vi "STAGE+mono+counter_edit17.vi"() -> ()   [LabVIEW 2017]
panel:
  out "XY Graph 2":cluster{"Y":dbl[], "Y":dbl[]}[](graph)
  out "Waveform Graph 2":waveform(dbl)[](graph)
  out "Waveform Graph":waveform(dbl)[](graph)
  out "XY Graph":cluster{dbl[], dbl[]}(graph)
  out "PROGRESS":u8(slide) max=10 step=10 scale=0.0..5.0
  in  "?":enum32{"DELAY", "COUNTER", "MONO", "PLOT"}(tab)
  out "Final time [ps]":dbl
  out "Current time [ps]":dbl
  out "Initial time [ps]":dbl
  in  "Set this as t0":bool
  in  "Axis":i32=1
  in  "Motor ON":bool
  in  "Motor OFF":bool
  out "Current Position [mm]":dbl
  out "Final Position [mm]":dbl
  in  "Data Points":i32=100
  out "Current Point":i32
  in  "Step Size [um]":i32=10
  in  "Target [mm]":dbl format="%.3f"
  in  "Move":bool
  out "Initial position [mm]":dbl
  in  "GPIB address":string="23"
  in  "Count Mode":u16(ring) items=["A,B for Preset T", "A-B for Preset T", "A+B for Preset T", "A for Preset B"]
  in  "Trigger mode":u16(ring) items=["10 MHz"=0, "Input 2"=2, "Input T"=3]
  in  "Channel A Input":u16(ring)=1 items=["10 MHz", "Input 1"]
  in  "Channel B Input":u16(ring)=2 items=["Input 1"=1, "Input 2"=2]
  in  "Number of Measurements\n to take at one point/ Number of Periods":u16=1 min=1 max=2000 step=1
  in  "Time between measurements\n at one point (s)/Dwell Time":dbl=0.002 min=0.002 max=60.0 step=0.001
  in  "gate mode (CW:0)":i16(slide) scale=0.0..2.0 scale format="%.2f"
  out "Counts":i32
  in  "Integrating time \nin 10^-7 sec":dbl=10000000.0
  in  "Discriminator Level (mV)":dbl min=-300.0 max=300.0 step=0.2
  in  "Discriminator Slope":bool
  in  "Channel":i16 min=0 max=2 step=1
  out "Grating #":dbl
  out "Blaze angle":dbl
  out "Grooves/mm":dbl
  out "Mono port":T1(ring)
  out "Time delay":u32=450000 min=1
  in  "Step size":dbl=10.0 min=0.0
  in  "Scan to":i32=4000
  in  "Scan from":i32=2600
  out "Current wavelength":dbl
  in  "?":bool
  in  "Array":dbl[](array[numeric])
  out "Numeric":i32
  out "Numeric 2":i32
  out "Timeout 2":bool
  in  "?":bool
  out "Timeout":bool
  in  "Collect Data!":bool
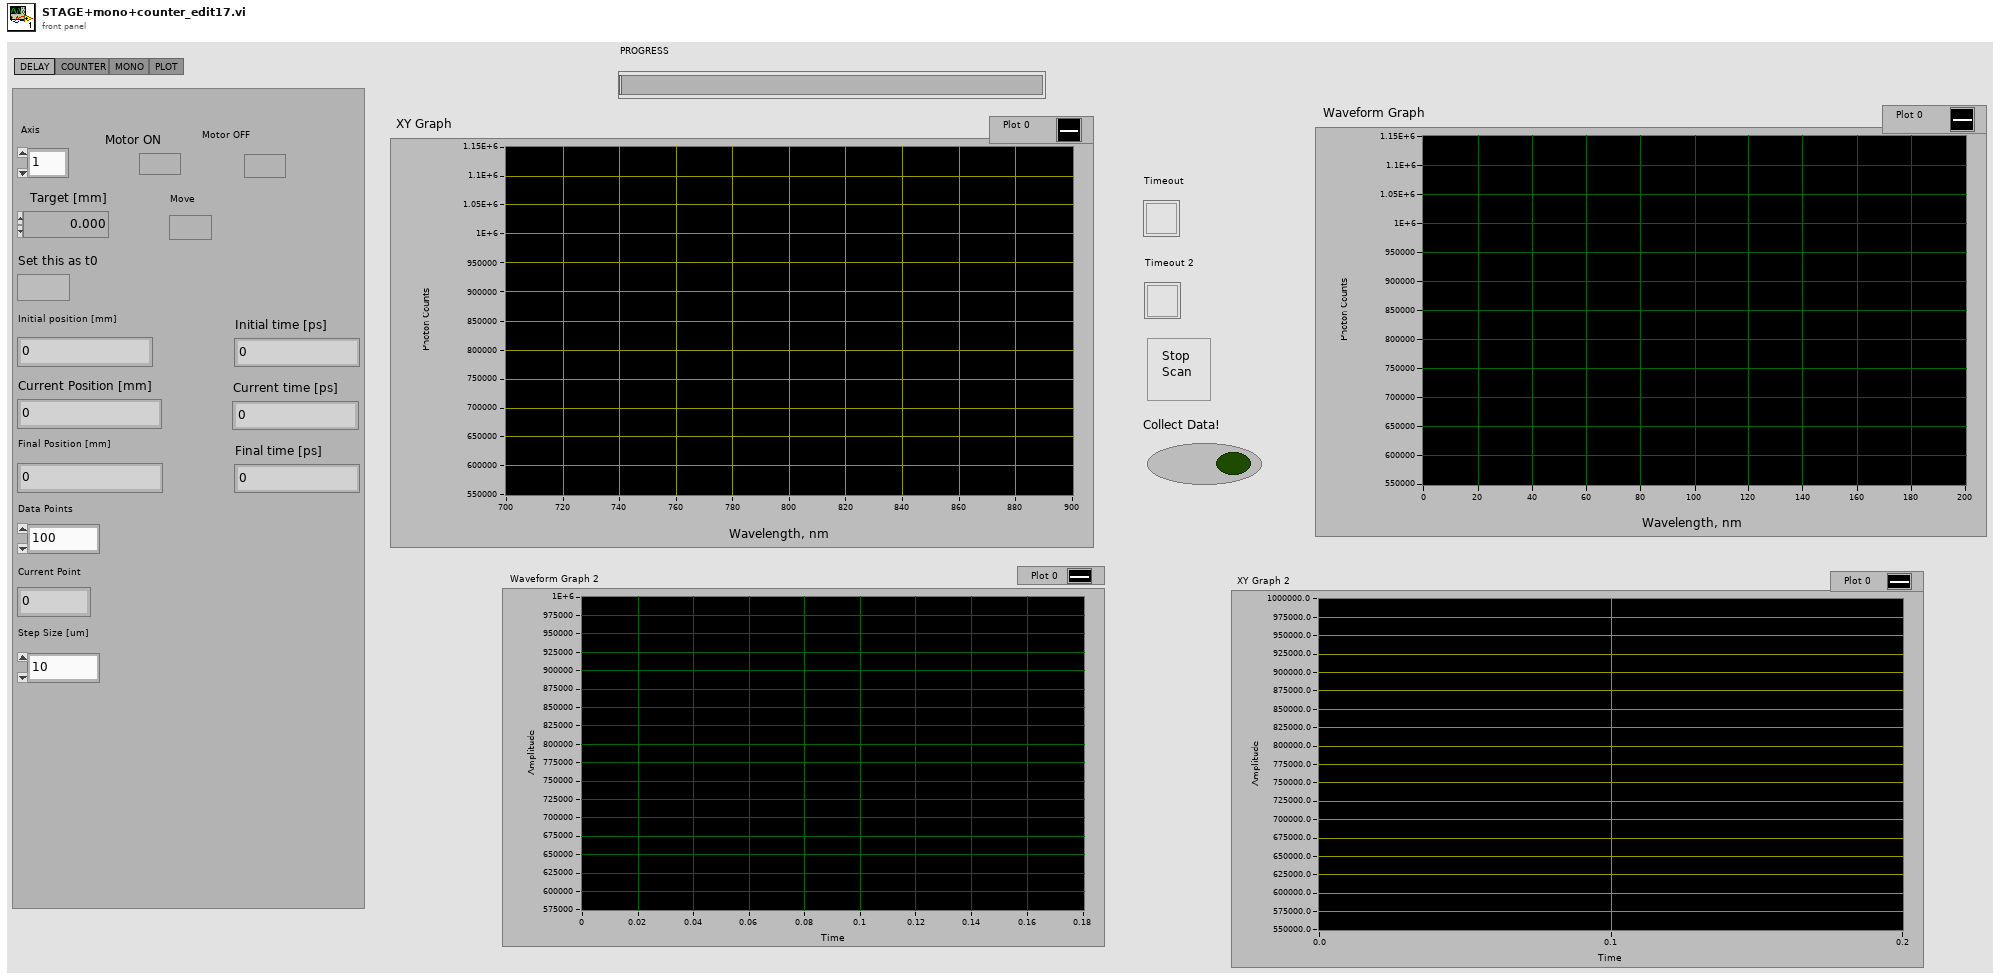
[diagram p1: front panel]
types:
  T1 = enum8{"COM 1", "COM 2", "COM 3", "COM 4", "COM 5", "COM 6", "COM 7", "COM 8", "COM 9"}
  T2 = cluster{"input XON/XOFF":bool, "input HW Handshake":bool, "input alt HW HShk":bool, "output XON/XOFF":bool, "output HW Handshake":bool, "output alt HW HShk":bool, "XOFF byte":u8, "XON byte":u8, "parity error byte":u16}
  T3 = enum16{"no parity", "odd parity", "even parity", "mark parity", "space parity"}
  T4 = typedef "NI_Matrix.lvlib/RealMatrix.ctl" = dbl[][]
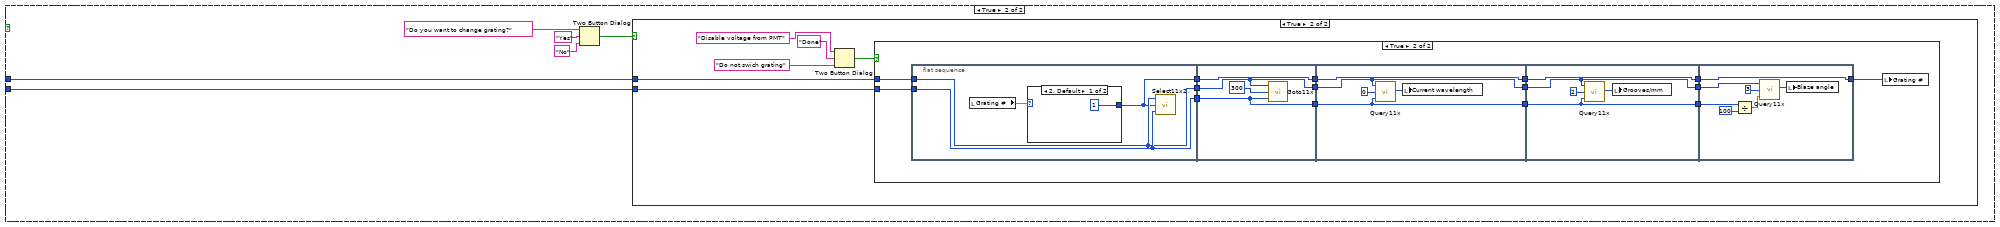
[diagram p2: hidden frame]
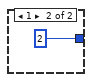
[diagram p5: hidden frame]
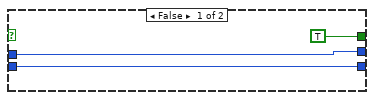
[diagram p6: hidden frame]
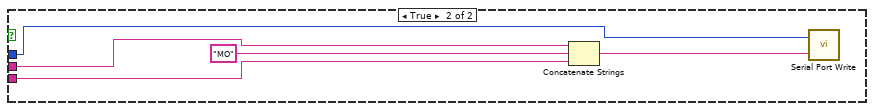
[diagram p7: hidden frame]
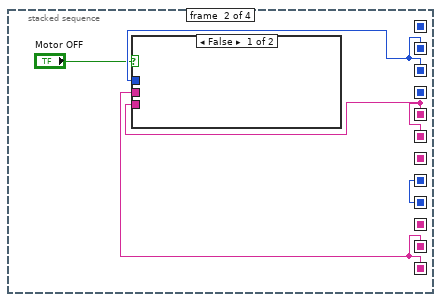
[diagram p8: hidden frame]
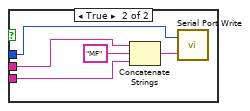
[diagram p9: hidden frame]
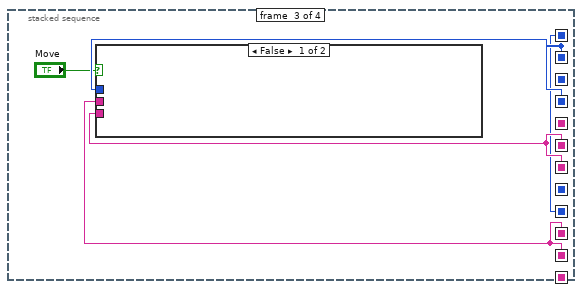
[diagram p10: hidden frame]
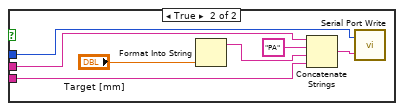
[diagram p11: hidden frame]
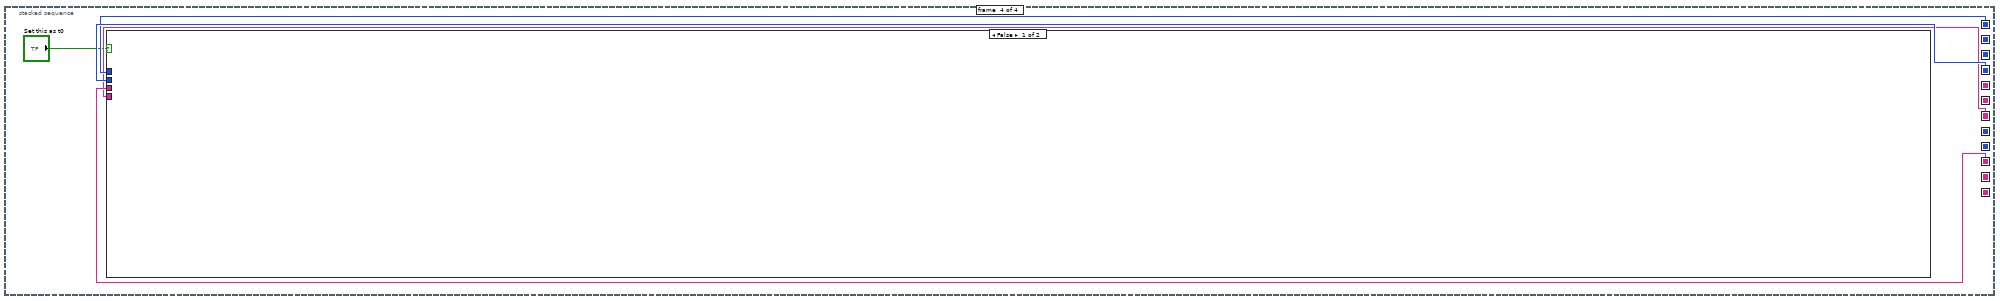
[diagram p12: hidden frame]
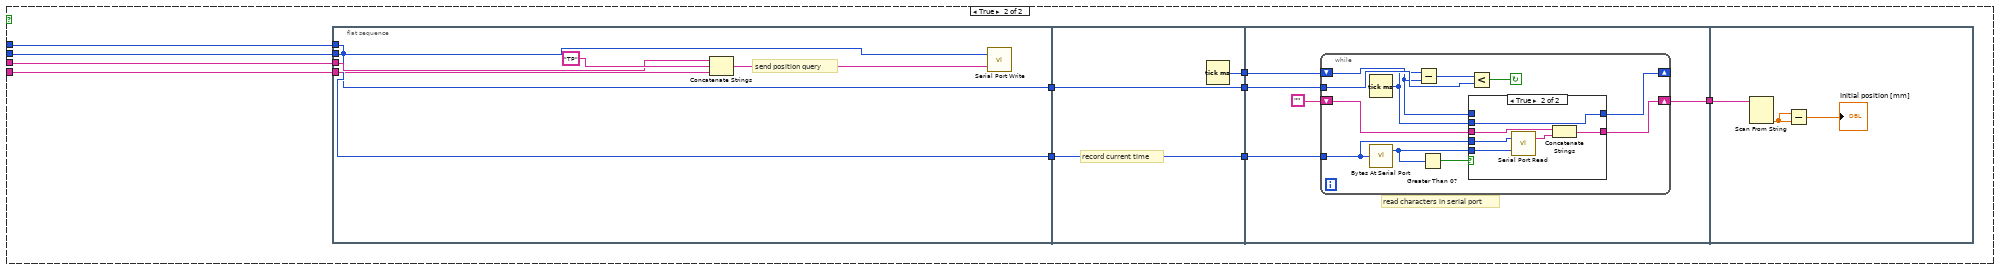
[diagram p13: hidden frame]
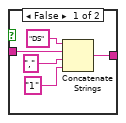
[diagram p15: hidden frame]
diagram:
  (unwired) FALSE
  w39 = u32 19200  # baud rate
  w38 = u16 8  # data bits
  w37 = enum16{"1 bit", "1.5 bits", "2 bits"}."1 bit"  # stop bits
  w41 = T3."no parity"  # parity
  w36 = 4  # 0=COM1 so n=COM(n+1)
  w40 = u16 1024  # buffer size
  n1 = flat-sequence {
    tunnel: ["Data Points"] -> w45
    tunnel: "Axis" -> [w67]
    tunnel: [w59] -> w44
    tunnel: [w67] -> w43
    tunnel: ["Step Size [um]"] -> w17
    tunnel: [w59] -> w16
    tunnel: ["Step Size [um]"] -> w15
    tunnel: ["Data Points"] -> w14
    tunnel: [w59] -> w13
    tunnel: [w58] -> w12
    tunnel: [w59] -> w10
    tunnel: [w58] -> w9
    tunnel: [w61] -> w8
    tunnel: [w51] -> w7
    tunnel: w45 -> [w155]
    tunnel: w44 -> [w154]
    tunnel: w43 -> [w153]
    tunnel: w36 -> [w149]
    tunnel: "GPIB address" -> [w148]
    tunnel: "GPIB address" -> [w147]
    tunnel: w17 -> [w136]
    tunnel: w16 -> [w134]
    tunnel: w15 -> [w133]
    tunnel: w14 -> [w131]
    tunnel: w13 -> [w126]
    tunnel: w12 -> [w125]
    tunnel: "Integrating time \nin 10^-7 sec" -> [w124]
    tunnel: w10 -> [w122]
    tunnel: w9 -> [w121]
    tunnel: w8 -> [w120]
    tunnel: w7 -> [w118]
    tunnel: w3 -> [w107]
    tunnel: w2 -> [w106]
    tunnel: w1 -> [w105]
    frame #0 {
      n2 = while {
        stop <- "Collect Data!" stop-if-true
        n3 = Multiply(x=1, y=1000) -> (x*y=w49:i32)
        n4 = Wait (ms)(milliseconds to wait=w49) -> ()  [unwired: 1 out]
      }
    }
    frame #1 {
      w52 = 1000000000000.0
      w57 = 1000
      w60 = 300000000
      w62 = 1000
      n5 = local read "Initial position [mm]"() -> (w59:dbl)
      n6 = Multiply(x="Step Size [um]", y="Data Points") -> (x*y=w66:i32)
      n7 = Divide(x="Step Size [um]", y=w62) -> (x/y=w61:dbl)
      n8 = Divide(x=w66, y=w62) -> (x/y=w65:dbl)
      n9 = Add(x=w59, y=w65) -> (x+y=w58:dbl)
      "Final Position [mm]" <- w58
      n10 = Divide(x=w58, y=w57) -> (x/y=w56:dbl)
      n11 = Divide(x=w59, y=w57) -> (x/y=w55:dbl)
      n12 = Divide(x=w56, y=w60) -> (x/y=w53:dbl)
      n13 = Divide(x=w55, y=w60) -> (x/y=w54:dbl)
      n14 = Multiply(x=w53, y=w52) -> (x*y=→"Final time [ps]":dbl)
      n15 = Multiply(x=w54, y=w52) -> (x*y=w51:dbl)
      "Initial time [ps]" <- w51
    }
    frame #2 {
      w87 = "\r\n"
      n16 = Increment(x=w131) -> (x+1=w132:i32)
      n17 = Divide(x=w136, y=1000.0) -> (x/y=w112:dbl)
      n18 = for {
        N: w132 -> [_]
        tunnel: w112 -> [w166]
        tunnel: w134 -> [w164]
        tunnel: [w157] -> w130 mode=indexing
        i -> [w165]
        # "distances"
        n19 = Multiply(x=w166, y=w165) -> (x*y=w163:dbl)
        n20 = Add(x=w164, y=w163) -> (x+y=w162:dbl)
        n21 = Divide(x=w162, y=1000) -> (x/y=w156:dbl)
        n22 = Divide(x=w156, y=300000000) -> (x/y=w159:dbl)
        n23 = Multiply(x=w159, y=1000000000000.0) -> (x*y=w157:dbl)
      }
      n24 = To Time Stamp(1:"Scan from") -> (0:w78:timestamp)
      n25 = Multiply(x="Scan to", y=1) -> (x*y=w119:i32)
      n26 = Multiply(x=1, y="Scan from") -> (x*y=w111:i32)
      n27 = Divide(x=w112, y=1000.0) -> (x/y=w113:dbl)
      n28 = Subtract(x=w119, y=w111) -> (x-y=w142:i32)
      n29 = local read "Initial time [ps]"() -> (w71:dbl)
      n30 = Divide(x=w142, y="Step size") -> (x/y=w141:dbl)
      n31 = Divide(x=w113, y=300000000) -> (x/y=w115:dbl)
      n32 = Bundle By Name("Y"=dbl[] [], "t0"=w78, "dt"="Step size") -> (w75:waveform(dbl))  [unwired: 1 in]
      n33 = To Time Stamp(1:w71) -> (0:w70:timestamp)
      n34 = Multiply(x=w115, y=1000000000000.0) -> (x*y=w69:dbl)
      n35 = Build Array(w75) -> (w74:waveform(dbl)[])
      n36 = Build Array(w118) -> (w108:dbl[])
      n37 = Round Toward -Infinity(1:w141) -> (0:w140:dbl)
      n38 = Concatenate Strings("\r", "\n") -> (w150:string)
      n39 = Bundle By Name("Y"=dbl[] [], "dt"=w69, "t0"=w70) -> (w73:waveform(dbl))  [unwired: 1 in]
      n40 = Build Array(w73) -> (w68:waveform(dbl)[])
      n41 = for {
        N: w155 -> [w223]
        tunnel: w154 -> [w250]
        tunnel: w133 -> [w246]
        tunnel: w153 -> [w243]
        tunnel: w150 -> [w240]
        tunnel: w149 -> [w241]
        tunnel: w148 -> [w239]
        tunnel: w106 -> [w236]
        tunnel: w107 -> [w238]
        tunnel: w147 -> [w237]
        tunnel: [w193] -> w80 mode=indexing
        tunnel: w111 -> [w231]
        tunnel: "Step size" -> [w230]
        tunnel: w140 -> [w229]
        tunnel: w126 -> [_]
        tunnel: w125 -> [_]
        tunnel: w124 -> [w228]
        tunnel: "Scan to" -> [w227]
        tunnel: "Scan from" -> [w226]
        tunnel: "Step size" -> [w201]
        tunnel: w122 -> [w218]
        tunnel: w121 -> [w216]
        tunnel: w120 -> [w219]
        tunnel: w69 -> [w185]
        tunnel: w118 -> [w224]
        tunnel: "Scan from" -> [w202]
        tunnel: "Step size" -> [w203]
        shift-right: [w177] -> _
        shift-left: w108 -> [w199]
        tunnel: w107 -> [w198]
        tunnel: w106 -> [w197]
        tunnel: w105 -> [w196]
        shift-right: [w190] -> _
        shift-left: w74 -> [w191]
        shift-right: [w180] -> _
        shift-left: w68 -> [w182]
        i -> [w206]
        w195 = dbl[] []
        w217 = 1000
        w220 = 300000000
        n42 = To Time Stamp(1:w231) -> ()  [unwired: 1 out]
        n43 = property on="PROGRESS" class="Slide (strict)"("Scale.Increment"=1, "Scale.Maximum"=w223, "Scale.Minimum"=0) -> ()  [unwired: 2 in, 2 out]
        n44 = flat-sequence {
          tunnel: w239 -> [w268]
          tunnel: w238 -> [w267]
          tunnel: w236 -> [w266]
          tunnel: w231 -> [w265]
          tunnel: w230 -> [w264]
          tunnel: w229 -> [w263]
          tunnel: w227 -> [w262]
          tunnel: w226 -> [w261]
          tunnel: w195 -> [w260]
          tunnel: w195 -> [w259]
          tunnel: w203 -> [w258]
          tunnel: w202 -> [w257]
          tunnel: w201 -> [w256]
          tunnel: w198 -> [w255]
          tunnel: w197 -> [w254]
          tunnel: w196 -> [w253]
          tunnel: [w251] -> w194
          tunnel: [w252] -> _
          tunnel: [w251] -> w192
          tunnel: [w432] -> w193
          tunnel: w194 -> [w432]
          tunnel: [w431] -> w175
          frame #0 {
            # "step size"
            n45 = while {
              tunnel: w266 -> [_]
              tunnel: w267 -> [_]
              tunnel: w268 -> [w274]
              tunnel: w265 -> [w302]
              tunnel: w264 -> [w301]
              tunnel: w263 -> [w300]
              tunnel: w262 -> [w270]
              tunnel: w261 -> [w269]
              tunnel: w256 -> [w271]
              tunnel: w258 -> [w298]
              shift-right: [w294] -> w251
              shift-left: w259 -> [w293]
              shift-right: [w288] -> w252
              shift-left: w260 -> [w296]
              tunnel: w257 -> [w291]
              tunnel: w255 -> [w278]
              tunnel: w254 -> [w277]
              tunnel: w253 -> [w276]
              i -> [w299]
              stop <- w305 stop-if-true
              n46 = property on="XY Graph" class="XYGraph (strict)"("XScale.Increment"=w271, "XScale.Maximum"=w270, "XScale.Minimum"=w269) -> ()  [unwired: 2 in, 2 out]
              n47 = property on="Waveform Graph" class="WFGraph (strict)"("XScale.Increment"=w271, "XScale.Maximum"=w270, "XScale.Minimum"=w269) -> ()  [unwired: 2 in, 2 out]
              n48 = Multiply(x=w299, y=w301) -> (x*y=w306:dbl)
              n49 = Multiply(x=w299, y=w298) -> (x*y=w297:dbl)
              n50 = Greater Or Equal?(x=w299, y=w300) -> (x >= y?=w303:bool)
              n51 = Add(x=w297, y=w291) -> ()  [unwired: 1 out]
              n52 = Add(x=w306, y=w302) -> (x+y=w275:dbl)
              n53 = Or(x="?", y=w303) -> (x .or. y?=w305:bool)
              n54 = Build Array (concatenate)(w296, w275) -> (w295:dbl[])
              n55 = flat-sequence {
                tunnel: w274 -> [w321]
                tunnel: w275 -> [w322]
                tunnel: [w322] -> w282
                tunnel: [w308] -> w281
                tunnel: [w307] -> w280
                tunnel: [w321] -> w279
                tunnel: w278 -> [w311]
                tunnel: w277 -> [w310]
                tunnel: w276 -> [w309]
                tunnel: [w355] -> w287
                tunnel: [w354] -> w286
                tunnel: [w352] -> w285
                tunnel: w282 -> [w356]
                tunnel: w281 -> [w355]
                tunnel: w280 -> [w354]
                tunnel: w279 -> [w352]
                tunnel: w287 -> [w363]
                tunnel: w286 -> [w362]
                tunnel: w285 -> [w357]
                tunnel: [w357] -> w273
                tunnel: w273 -> [w365]
                tunnel: [w365] -> w272
                tunnel: w272 -> [w418]
                tunnel: [w418] -> w284
                tunnel: w284 -> [w419]
                tunnel: [w419] -> w283
                tunnel: [w425] -> w290
                tunnel: w283 -> [w426]
                frame #0 {
                  n56 = flat-sequence {
                    tunnel: w311 -> [w328]
                    tunnel: [w328] -> w320
                    tunnel: w310 -> [w330]
                    tunnel: [w330] -> w319
                    tunnel: w309 -> [w326]
                    tunnel: [w326] -> w318
                    tunnel: w320 -> [w334]
                    tunnel: [w334] -> w317
                    tunnel: w319 -> [w335]
                    tunnel: [w335] -> w316
                    tunnel: w318 -> [w332]
                    tunnel: [w332] -> w315
                    tunnel: w317 -> [w343]
                    tunnel: [w343] -> w314
                    tunnel: w316 -> [w340]
                    tunnel: [w340] -> w313
                    tunnel: w315 -> [w338]
                    tunnel: [w338] -> w312
                    tunnel: w314 -> [w345]
                    tunnel: w313 -> [w346]
                    tunnel: w312 -> [_]
                    tunnel: [w346] -> w308
                    tunnel: [w345] -> w307
                    frame #0 {
                      n57 = call "Query11x.vi"("port number"=w330, "QUERY"=u16 0, "time delay"=w328) -> ("timeout"=w327:bool, "STATUS MESSAGE"=w325:u16)  [unwired: 2 out]
                      n58 = local write "Timeout"(w327) -> ()
                      n59 = Divide(x=w325, y=1 ("Numeric")) -> (x/y=→"Current wavelength":dbl)
                    }
                    frame #1 {
                      n60 = call "Query11x.vi"("port number"=w335, "QUERY"=u16 2, "time delay"=w334) -> ("timeout"=w333:bool, "STATUS MESSAGE"=→"Grooves/mm":u16)  [unwired: 2 out]
                      n61 = local write "Timeout"(w333) -> ()
                    }
                    frame #2 {
                      n62 = Divide(x=w343, y=i16 100 ("device (1)")) -> (x/y=w341:dbl)
                      n63 = call "Query11x.vi"("port number"=w340, "QUERY"=u16 3, "time delay"=w341) -> ("timeout"=w339:bool, "STATUS MESSAGE"=→"Blaze angle":u16)  [unwired: 2 out]
                      n64 = local write "Timeout"(w339) -> ()
                    }
                    frame #3 {
                      n65 = Divide(x=w345, y=i16 100 ("device (1)")) -> (x/y=w349:dbl)
                      n66 = call "Query11x.vi"("port number"=w346, "QUERY"=u16 4, "time delay"=w349) -> ("timeout"=w348:bool, "STATUS MESSAGE"=→"Grating #":u16)  [unwired: 2 out]
                      n67 = local write "Timeout"(w348) -> ()
                    }
                  }
                }
                frame #1 {
                  n68 = call "Goto11x.vi"("time delay"=w354, "WAVELENGTH"=w356, "port number"=w355) -> ("timeout"=w353:bool)  [unwired: 2 out]
                  n69 = local write "Timeout 2"(w353) -> ()
                }
                frame #2 {
                  # "set counter time in 10^-7 seconds in CW"
                  n70 = call "Query11x.vi"("port number"=w363, "QUERY"=0, "time delay"=w362) -> ("timeout"=w361:bool, "STATUS MESSAGE"=w360:u16)  [unwired: 2 out]
                  n71 = local write "Timeout 2"(w361) -> ()
                  n72 = Divide(x=w360, y=1) -> (x/y=w359:dbl)
                  n73 = local write "Current wavelength"(w359) -> ()
                }
                frame #3 {
                  # "Configures discriminator."
                  n74 = flat-sequence {
                    tunnel: w365 -> [w375]
                    tunnel: [w375] -> w374
                    tunnel: [w382] -> w373
                    tunnel: [w380] -> w372
                    tunnel: "Discriminator Slope" -> [w381]
                    tunnel: w374 -> [w380]
                    tunnel: w366 -> [w379]
                    tunnel: w373 -> [w401]
                    tunnel: [w402] -> w371
                    tunnel: w372 -> [w400]
                    tunnel: [w400] -> w370
                    tunnel: w366 -> [w398]
                    tunnel: w371 -> [w414]
                    tunnel: w370 -> [w413]
                    tunnel: "Discriminator Level (mV)" -> [w408]
                    tunnel: w366 -> [w407]
                    frame #0 {
                      # "Flush I/O buffers."
                      n75 = for {
                        N: 5 -> [_]
                        tunnel: w375 -> [w377]
                        n76 = GPIB Write(0:w377, 1:"\r") -> ()  [unwired: 3 in, 2 out]
                      }
                    }
                    frame #1 {
                      # "Set discriminator slope."
                      n77 = case shown="True" w381 {
                        tunnel: [w388 w393] -> w383
                        tunnel: w379 -> [w387 w392]
                        frame False {
                          n78 = Concatenate Strings("DS", w387, ",", "1") -> (w388:string)
                        }
                        frame True {
                          n79 = Concatenate Strings("DS", w392, ",", "0") -> (w393:string)
                        }
                      }
                      n80 = GPIB Write(0:w380, 1:w383, 2:5) -> (6:w382:errorcluster)  [unwired: 2 in, 1 out]
                    }
                    frame #2 {
                      # "Set discriminator mode to fixed."
                      n81 = Concatenate Strings("DM", w398, ",", "0") -> (w397:string)
                      n82 = GPIB Write(0:w400, 1:w397, 2:5, 3:w401) -> (6:w402:errorcluster)  [unwired: 1 in, 1 out]
                    }
                    frame #3 {
                      # "Set discriminator level.\nMust be between +300 and -300 mV."
                      n83 = Divide(x=w408, y=1000.0) -> (x/y=w416:dbl)
                      n84 = Number To Fractional String(number=w416, precision (6)=i16 4) -> (F-format string=w405:string)  [unwired: 2 in]
                      n85 = Concatenate Strings("DL", w407, ",", w405) -> (w412:string)
                      n86 = GPIB Write(0:w413, 1:w412, 2:5, 3:w414) -> (6:w409:errorcluster)  [unwired: 1 in, 1 out]
                      n87 = call <vilib>:"General Error Handler.vi"("type of dialog (OK msg:1)"=1, "error in (no error)"=w409) -> ()  [unwired: 9 in, 5 out]
                    }
                  }
                  n88 = Number To Decimal String(number="Channel") -> (decimal integer string=w366:string)  [unwired: 1 in]
                }
                frame #4 {
                  n89 = call "Start.vi"("GPIB Address"=w418) -> ()  [unwired: 9 in]
                }
                frame #5 {
                  # "Wait for Scan to Finish"
                  n90 = for {
                    N: 1 -> [_]
                    tunnel: w419 -> [w421]
                    n91 = while {
                      tunnel: w421 -> [w422]
                      stop <- w424 stop-if-true
                      n92 = call "ScanDone.vi"("Wait (ms)"=1000, "GPIB Address"=w422) -> ("Scan Finished?"=w424:bool)
                    }
                  }
                }
                frame #6 {
                  n93 = call "Read Data.vi"("Channel Number"=0, "GPIB Address"=w426, "Number of Datapoints"=1) -> ("Data"=w427:i32[])
                  n94 = Index Array(array=w427, index=0) -> (element=w425:i32)
                  "Counts" <- w425
                }
              }
              n95 = Build Array (concatenate)(w293, w290) -> (w292:dbl[])
              n96 = Bundle(w295, w292) -> (w289:cluster{dbl[], dbl[]})  [unwired: 1 in]
              "XY Graph" <- w289
              n97 = Unbundle(w289) -> (w288:dbl[], w294:dbl[])
            }
          }
          frame #1 {
            n98 = Array Size(array="Array") -> (size(s)=w433:i32)
            n99 = flat-sequence {
              tunnel: w432 -> [w439]
              tunnel: "Array" -> [w438]
              tunnel: w433 -> [w437]
              tunnel: [w435] -> w431
              frame #0 {
                n100 = for {
                  N: w437 -> [w444]
                  tunnel: w438 -> [w451]
                  tunnel: w439 -> [w446]
                  shift-right: [w440] -> w435
                  shift-left: dbl[] [] -> [w441]
                  i -> [w443]
                  n101 = local read "Scan from"() -> (w449:i32)
                  n102 = Index Array(array=w451, index=w443) -> (element=w450:dbl)
                  n103 = local read "Step size"() -> (w447:dbl)
                  n104 = Subtract(x=w450, y=w449) -> (x-y=w448:dbl)
                  n105 = Divide(x=w448, y=w447) -> (x/y=w445:dbl)
                  n106 = Index Array(array=w446, index=w445) -> (element=w442:dbl)
                  n107 = Insert Into Array(array=w441, index=w443, new element=w442) -> (w440:dbl[])
                  "Numeric" <- w444
                }
              }
            }
          }
        }
        n108 = stacked-sequence {
          tunnel: w236 -> [w453]
          tunnel: w237 -> [_]
          frame #0 {
            n109 = call <vilib>:"Close Serial Driver.vi"("port number"=w453) -> ()  [unwired: 1 out]
            n110 = GPIB Misc(0:"loc 23" ("command string")) -> ()  [unwired: 1 in, 3 out]
          }
        }
        n111 = Divide(x=w219, y=w217) -> (x/y=w215:dbl)
        n112 = Divide(x=w216, y=w217) -> (x/y=w213:dbl)
        n113 = Divide(x=w218, y=w217) -> (x/y=w214:dbl)
        n114 = Multiply(x=w185, y=w206) -> (x*y=w225:dbl)
        n115 = Number To Decimal String(number=w228) -> (decimal integer string=w234:string)  [unwired: 1 in]
        n116 = Add(x=1, y=w206) -> (x+y=→"PROGRESS":i32)
        n117 = Divide(x=w246, y=1000) -> (x/y=w245:dbl)
        n118 = Divide(x=w215, y=w220) -> (x/y=w209:dbl)
        n119 = Divide(x=w213, y=w220) -> (x/y=w207:dbl)
        n120 = Divide(x=w214, y=w220) -> (x/y=w208:dbl)
        n121 = Add(x=w224, y=w225) -> (x+y=w200:dbl)
        n122 = Concatenate Strings("CP 2,", w234) -> (w232:string)
        n123 = Multiply(x=w209, y=1000000000000.0) -> (x*y=w174:dbl)
        n124 = Multiply(x=w207, y=1000000000000.0) -> (x*y=w173:dbl)
        n125 = Multiply(x=w208, y=1000000000000.0) -> (x*y=w172:dbl)
        n126 = Multiply(x=w245, y=w206) -> (x*y=w249:dbl)
        n127 = Build Array (concatenate)(w199, w200) -> (w177:dbl[])
        n128 = Add(x=w250, y=w249) -> (x+y=w248:dbl)
        n129 = Format Into String(w243) -> (resulting string=w242:string)  [unwired: 3 in, 1 out]
        n130 = GPIB Write(0:w239, 1:w232, 2:i16 5 ("mode (0)")) -> ()  [unwired: 2 in, 2 out]
        n131 = flat-sequence {
          tunnel: w248 -> [w456]
          tunnel: [w456] -> w244
          tunnel: w240 -> [w458]
          tunnel: w242 -> [w457]
          tunnel: w241 -> [w454]
          tunnel: w244 -> [w467]
          frame #0 {
            n132 = Format Into String(w456) -> (resulting string=w455:string)  [unwired: 3 in, 1 out]
            n133 = Wait (ms)(milliseconds to wait=u32 100) -> ()  [unwired: 1 out]
            n134 = Concatenate Strings(w457, "PA" ("Substring"), w455, w458) -> (w460:string)
            n135 = call <vilib>:"Serial Port Write.vi"("string to write"=w460, "port number"=w454) -> ()  [unwired: 1 out]
          }
          frame #1 {
            n136 = Divide(x=w467, y=1000) -> (x/y=w465:dbl)
            n137 = Wait (ms)(milliseconds to wait=u32 1000) -> ()  [unwired: 1 out]
            n138 = Divide(x=w465, y=300000000) -> (x/y=w464:dbl)
            n139 = Multiply(x=w464, y=1000000000000.0) -> (x*y=→"Current time [ps]":dbl)
            "Current Position [mm]" <- w467
          }
        }
        n140 = property on="Waveform Graph 2" class="WFGraph (strict)"("XScale.Increment"=w174, "XScale.Maximum"=w173, "XScale.Minimum"=w172) -> ()  [unwired: 2 in, 2 out]
        n141 = property on="XY Graph 2" class="XYGraph (strict)"("XScale.Increment"=w174, "XScale.Maximum"=w173, "XScale.Minimum"=w172) -> ()  [unwired: 2 in, 2 out]
        n142 = local read "Scan from"() -> (w188:i32)
        n143 = local read "Step size"() -> (w186:dbl)
        n144 = To Time Stamp(1:w188) -> (0:w187:timestamp)
        n145 = Bundle By Name("Y"=w192, "t0"=w187, "dt"=w186) -> (w189:waveform(dbl))  [unwired: 1 in]
        n146 = Build Array (concatenate)(w191, w189) -> (w190:waveform(dbl)[])
        "Waveform Graph" <- w190
        n147 = local read "Initial time [ps]"() -> (w184:dbl)
        n148 = To Time Stamp(1:w184) -> (0:w183:timestamp)
        n149 = call "Convert to Dynamic Data"("Array"=w177) -> ("Dynamic Data Type"=w179:dynamicdata)  [unwired: 3 in]
        n150 = Bundle By Name("Y"=w175, "t0"=w183, "dt"=w185) -> (w181:waveform(dbl))  [unwired: 1 in]
        n151 = call "Convert to Dynamic Data2"("Array"=w175) -> ("Dynamic Data Type"=w176:dynamicdata)  [unwired: 3 in]
        n152 = call "Build XY Graph"("Y Input"=w176, "X Input"=w179) -> ("XY Graph"=→"XY Graph 2":cluster{"X":dbl[], "Y":dbl[]}[])  [unwired: 8 in, 1 out]
        n153 = Build Array (concatenate)(w182, w181) -> (w180:waveform(dbl)[])
        "Waveform Graph 2" <- w180
        "Current Point" <- w206
        "Numeric 2" <- w223
      }
      n154 = Increment(x=w140) -> (x+1=w110:dbl)
      n155 = for {
        N: w110 -> [_]
        tunnel: "Step size" -> [w171]
        tunnel: w111 -> [w169]
        tunnel: [w167] -> w109 mode=indexing
        i -> [w170]
        # "wavelengths"
        n156 = Multiply(x=w171, y=w170) -> (x*y=w168:dbl)
        n157 = Add(x=w169, y=w168) -> (x+y=w167:dbl)
      }
      n158 = Build Array (concatenate)(0, w130) -> (w81:dbl[])
      n159 = Build Array(w109) -> (w139:dbl[][])
      n160 = local read "Integrating time \nin 10^-7 sec"() -> (w85:dbl)
      n161 = Transpose Matrix(1:w139) -> (0:w138:dbl[][])
      n162 = Transpose Matrix(1:w80) -> (0:w137:dbl[][])
      n163 = Build Array (concatenate)(w138, w137) -> (w82:T4)
      n164 = Insert Into Array(array=w82, index (row)=0, new element=w81) -> (w127:T4)  [unwired: 1 in]
      n165 = local read "Blaze angle"() -> (w104:dbl)
      n166 = local read "Grating #"() -> (w103:dbl)
      n167 = Multiply(x=w85, y=1e-07) -> (x*y=w84:dbl)
      n168 = Get Date/Time In Seconds() -> (seconds since 1Jan1904=w97:timestamp)
      n169 = Array To Spreadsheet String(delimiter (Tab)=",", array=w127, 3:"%f" ("format string")) -> (spreadsheet string=w86:string)
      n170 = Format Date/Time String(time format string (%c)="%Y-%b-%d %H:%M:%S", seconds (now)=w97) -> (date/time string=w98:string)  [unwired: 1 in]
      n171 = Number To Decimal String(number=w84) -> (decimal integer string=w99:string)  [unwired: 1 in]
      n172 = Number To Decimal String(number=w103) -> (decimal integer string=w100:string)  [unwired: 1 in]
      n173 = Number To Decimal String(number=w104) -> (decimal integer string=w88:string)  [unwired: 1 in]
      n174 = call <vilib>:"Space Constant.vi"() -> ("String"=w101:string)
      n175 = Concatenate Strings(w87, "Data was taken on ", w98, w87, "Integration Time is ", w99, w101, "s", w87, "Monochromator gratng # ", w100, "; ", "blazed for ", w88, w101, "nm", w87, w87, w87, w86) -> (w102:string)
      n176 = Write to Text File(text=w102) -> ()  [unwired: 3 in, 3 out]
    }
  }
  n177 = flat-sequence {
    tunnel: [w471] -> w30
    tunnel: [w470] -> w29
    frame #0 {
      n178 = call "CM Com Read ini.vi"() -> ("Mono port"=w470:T1, "time delay1"=w471:u32)  [unwired: 7 in]
    }
  }
  n179 = call <vilib>:"Serial Port Init.vi"("flow control etc."=T2 {"input XON/XOFF"=FALSE, "input HW Handshake"=FALSE, "input alt HW HShk"=FALSE, "output XON/XOFF"=FALSE, "output HW Handshake"=FALSE, "output alt HW HShk"=FALSE, "XOFF byte"=13, "XON byte"=11, "parity error byte"=0}, "parity"=w41, "buffer size"=w40, "stop bits"=w37, "data bits"=w38, "baud rate"=w39, "port number"=w36) -> ("error code"=w35:i32)
  n180 = call "CM Serial Port Setup.vi"("COM port"=w29, "time delay"=w30) -> ("time delay1"=w25:u32, "DK port Out"=w26:T1, "error code"=w28:i32)  [unwired: 7 in]
  n181 = Equal To 0?(x=w28) -> (x = 0?=w27:bool)
  n182 = Concatenate Strings("\r", "\n") -> (w31:string)
  n183 = while {
    tunnel: w36 -> [w474]
    tunnel: w31 -> [w475]
    tunnel: w35 -> [_]
    tunnel: "Axis" -> [w472]
    stop <- TRUE continue-if-true
    w473 = u32 200  # timeout
    n184 = Format Into String(w472) -> (resulting string=w476:string)  [unwired: 3 in, 1 out]
    n185 = stacked-sequence {
      seq-local: [w481 _ _ _] -> [_ w492 _ _]
      seq-local: [w480 _ _ _] -> [_ w491 _ _]
      seq-local: [w482 _ _ _] -> [_ w493 _ _]
      seq-local: [w479 _ _ _] -> [_ w489 _ _]
      seq-local: [_ w492 _ _] -> [_ _ w502 _]
      seq-local: [_ w491 _ _] -> [_ _ w501 _]
      seq-local: [_ w493 _ _] -> [_ _ w503 _]
      seq-local: [_ w489 _ _] -> [_ _ w499 _]
      seq-local: [_ _ w502 _] -> [_ _ _ w515]
      seq-local: [_ _ w501 _] -> [_ _ _ w512]
      seq-local: [_ _ w503 _] -> [_ _ _ w514]
      seq-local: [_ _ w499 _] -> [_ _ _ w513]
      tunnel: w476 -> [w481 _ _ _]
      tunnel: w475 -> [w480 _ _ _]
      tunnel: w474 -> [w482 _ _ _]
      tunnel: w473 -> [w479 _ _ _]
      frame #0 {
        n186 = case shown="False" "Motor ON" {
          tunnel: w482 -> [_ w488]
          tunnel: w481 -> [_ w485]
          tunnel: w480 -> [_ w484]
          frame False {
          }
          frame True {
            n187 = Concatenate Strings(w485, "MO" ("Substring"), w484) -> (w486:string)
            n188 = call <vilib>:"Serial Port Write.vi"("string to write"=w486, "port number"=w488) -> ()  [unwired: 1 out]
          }
        }
      }
      frame #1 {
        n189 = case shown="False" "Motor OFF" {
          tunnel: w493 -> [_ w498]
          tunnel: w492 -> [_ w495]
          tunnel: w491 -> [_ w494]
          frame False {
          }
          frame True {
            n190 = Concatenate Strings(w495, "MF" ("Substring"), w494) -> (w496:string)
            n191 = call <vilib>:"Serial Port Write.vi"("string to write"=w496, "port number"=w498) -> ()  [unwired: 1 out]
          }
        }
      }
      frame #2 {
        n192 = case shown="False" "Move" {
          tunnel: w503 -> [_ w510]
          tunnel: w502 -> [_ w507]
          tunnel: w501 -> [_ w506]
          frame False {
          }
          frame True {
            n193 = Format Into String("Target [mm]") -> (resulting string=w504:string)  [unwired: 3 in, 1 out]
            n194 = Concatenate Strings(w507, "PA" ("Substring"), w504, w506) -> (w508:string)
            n195 = call <vilib>:"Serial Port Write.vi"("string to write"=w508, "port number"=w510) -> ()  [unwired: 1 out]
          }
        }
      }
      frame #3 {
        n196 = case shown="False" "Set this as t0" {
          tunnel: w515 -> [_ w525]
          tunnel: w514 -> [_ w524]
          tunnel: w513 -> [_ w523]
          tunnel: w512 -> [_ w522]
          frame False {
          }
          frame True {
            n197 = flat-sequence {
              tunnel: w525 -> [w529]
              tunnel: w524 -> [w528]
              tunnel: [w528] -> w521
              tunnel: w523 -> [w526]
              tunnel: [w526] -> w520
              tunnel: w522 -> [w527]
              tunnel: w521 -> [w533]
              tunnel: [w533] -> w519
              tunnel: w520 -> [w532]
              tunnel: [w532] -> w518
              tunnel: [w534] -> w517
              tunnel: w519 -> [w539]
              tunnel: w518 -> [w537]
              tunnel: w517 -> [w536]
              tunnel: [w535] -> w516
              tunnel: w516 -> [w561]
              frame #0 {
                # "send position query"
                n198 = Concatenate Strings(w529, "TP" ("Substring"), w527) -> (w530:string)
                n199 = call <vilib>:"Serial Port Write.vi"("string to write"=w530, "port number"=w528) -> ()  [unwired: 1 out]
              }
              frame #1 {
                # "record current time"
                n200 = Tick Count (ms)() -> (millisecond timer value=w534:u32)
              }
              frame #2 {
                # "read characters in serial port"
                n201 = while {
                  shift-left: w536 -> [w540]
                  shift-right: [w541] -> _
                  tunnel: w537 -> [w544]
                  shift-left: "" -> [w547]
                  shift-right: [w546] -> w535
                  tunnel: w539 -> [w548]
                  stop <- w543 continue-if-true
                  n202 = Tick Count (ms)() -> (millisecond timer value=w542:u32)
                  n203 = call <vilib>:"Bytes At Serial Port.vi"("port number"=w548) -> ("byte count"=w549:u32)  [unwired: 1 out]
                  n204 = Subtract(x=w542, y=w540) -> (x-y=w545:u32)
                  n205 = Greater Than 0?(x=w549) -> (x > 0?=w550:bool)
                  n206 = case shown="True" w550 {
                    tunnel: w549 -> [_ w558]
                    tunnel: w548 -> [_ w557]
                    tunnel: w547 -> [w552 w555]
                    tunnel: [w552 w554] -> w546
                    tunnel: [w551 w553] -> w541
                    tunnel: w542 -> [_ w553]
                    tunnel: w540 -> [w551 _]
                    frame False {
                    }
                    frame True {
                      n207 = call <vilib>:"Serial Port Read.vi"("requested byte count"=w558, "port number"=w557) -> ("string read"=w556:string)  [unwired: 1 out]
                      n208 = Concatenate Strings(w555, w556) -> (w554:string)
                    }
                  }
                  n209 = Less?(x=w545, y=w544) -> (x < y?=w543:bool)
                }
              }
              frame #3 {
                n210 = Scan From String(input string=w561) -> (output 1=w559:dbl)  [unwired: 4 in, 3 out]
                n211 = Subtract(x=w559, y=w559) -> (x-y=→"Initial position [mm]":dbl)
              }
            }
          }
        }
      }
    }
    n212 = Wait Until Next ms Multiple(millisecond multiple=u32 50) -> ()  [unwired: 1 out]
  }
  n213 = case shown="True" w27 {
    tunnel: w26 -> [w564 w567]
    tunnel: w25 -> [w563 w566]
    tunnel: [w564 w567] -> w2
    tunnel: [w563 w566] -> w3
    tunnel: [TRUE FALSE] -> w1
    frame False {
    }
    frame True {
      n214 = call "CM Com Write ini.vi"("time delay1"=w567, "Mono port"=w566) -> ()  [unwired: 7 in]
      n215 = local write "Mono port"(w567) -> ()
      n216 = local write "Time delay"(w566) -> ()
    }
  }
  n217 = call "Configure.vi"("Dwell Time (s)"="Time between measurements\n at one point (s)/Dwell Time", "Channel T Input"="Trigger mode", "Channel B Input"="Channel B Input", "Channel A Input"="Channel A Input", "Integrating time, 10^-7 sec"="Integrating time \nin 10^-7 sec", "gate mode (CW:0)"="gate mode (CW:0)", "Scan End Mode"=FALSE, "Number of Periods"="Number of Measurements\n to take at one point/ Number of Periods", "Count Mode"="Count Mode", "GPIB Address"="GPIB address") -> ()
  n218 = case shown="False" "?" {
    tunnel: w3 -> [_ w569]
    tunnel: w2 -> [_ w568]
    frame False {
    }
    frame True {
      n219 = Two Button Dialog(message="Do you want to change grating?", 1:"No" ("F button name (\"Cancel\")"), 2:"Yes" ("T button name (\"OK\")")) -> (T button?=w570:bool)
      n220 = case shown="True" w570 {
        tunnel: w569 -> [_ w575]
        tunnel: w568 -> [_ w574]
        frame False {
        }
        frame True {
          n221 = Two Button Dialog(message="Disable voltage from PMT", 1:"Do not swich grating" ("F button name (\"Cancel\")"), 2:"Done" ("T button name (\"OK\")")) -> (T button?=w576:bool)
          n222 = case shown="True" w576 {
            tunnel: w575 -> [_ w594]
            tunnel: w574 -> [_ w593]
            frame False {
            }
            frame True {
              n223 = flat-sequence {
                tunnel: w594 -> [w598]
                tunnel: [w598] -> w591
                tunnel: w593 -> [w597]
                tunnel: [w597] -> w590
                tunnel: [w595] -> w589
                tunnel: w591 -> [w602]
                tunnel: [w602] -> w588
                tunnel: w590 -> [w603]
                tunnel: [w603] -> w587
                tunnel: w589 -> [w601]
                tunnel: [w601] -> w586
                tunnel: w588 -> [w609]
                tunnel: [w609] -> w585
                tunnel: w587 -> [w608]
                tunnel: [w608] -> w584
                tunnel: w586 -> [w606]
                tunnel: [w606] -> w583
                tunnel: w585 -> [w612]
                tunnel: [w612] -> w582
                tunnel: w584 -> [w613]
                tunnel: [w613] -> w581
                tunnel: w583 -> [w611]
                tunnel: [w611] -> w580
                tunnel: w582 -> [w617]
                tunnel: w581 -> [w618]
                tunnel: [w616] -> w592
                tunnel: w580 -> [w616]
                frame #0 {
                  n224 = local read "Grating #"() -> (w596:dbl)
                  n225 = case shown="2, Default" w596 {
                    tunnel: [1 2] -> w595
                    frame 2, Default {
                    }
                    frame 1 {
                    }
                  }
                  n226 = call "Select11x2.vi"("time delay"=w598, "NEW GRT?"=w595, "port number"=w597) -> ()  [unwired: 3 out]
                }
                frame #1 {
                  n227 = call "Goto11x.vi"("time delay"=w602, "WAVELENGTH"=u16 300, "port number"=w603) -> ()  [unwired: 3 out]
                }
                frame #2 {
                  n228 = call "Query11x.vi"("port number"=w608, "QUERY"=u16 0, "time delay"=w609) -> ("STATUS MESSAGE"=w605:u16)  [unwired: 3 out]
                  n229 = local write "Current wavelength"(w605) -> ()
                }
                frame #3 {
                  n230 = call "Query11x.vi"("port number"=w613, "QUERY"=u16 2, "time delay"=w612) -> ("STATUS MESSAGE"=w610:u16)  [unwired: 3 out]
                  n231 = local write "Grooves/mm"(w610) -> ()
                }
                frame #4 {
                  n232 = Divide(x=w617, y=i16 100 ("device (1)")) -> (x/y=w619:dbl)
                  n233 = call "Query11x.vi"("port number"=w618, "QUERY"=u16 3, "time delay"=w619) -> ("STATUS MESSAGE"=w615:u16)  [unwired: 3 out]
                  n234 = local write "Blaze angle"(w615) -> ()
                }
              }
              n235 = local write "Grating #"(w592) -> ()
            }
          }
        }
      }
    }
  }
  "Mono port" <- w29
  "Time delay" <- w30
